vi "GSE 350 Read Data.vi"(8 "error in (no error)":errorcluster, 11 "VISA Refnum in":refnum<visa-resource-name>) -> (0 "error out":errorcluster, 2 "Raw Data":string, 3 "VISA Refnum out":refnum<visa-resource-name>)   [LabVIEW 2019]
uses:
  <vilib>/Utility/error.llb/whitespace.ctl
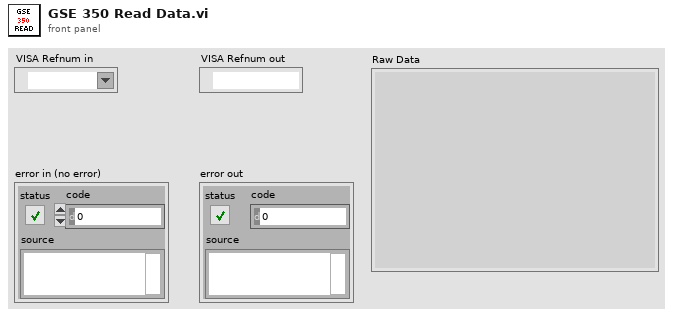
[diagram p1: front panel]
types:
  T1 = typedef "whitespace.ctl" = u16
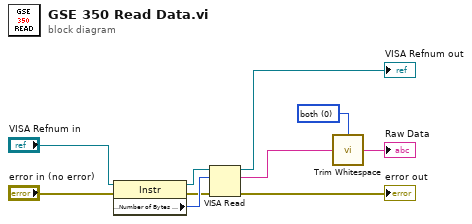
[diagram p0: block diagram]
diagram:
  w8 = T1 0 items=["both", "start of string", "end of string"] ("location (both)")
  n1 = property class="Instr"(reference="VISA Refnum in", error in="error in (no error)") -> (reference out=w4:refnum<visa-resource-name>, error out=w2:errorcluster, "Serial Settings:Number of Bytes at Serial Port"=w7:u32)
  n2 = VISA Read(VISA resource name=w4, byte count=w7, error in (no error)=w2) -> (VISA resource name out=→"VISA Refnum out":refnum<visa-resource-name>, read buffer=w9:string, error out=→"error out":errorcluster)  [unwired: 1 out]
  n3 = call <vilib>:"Trim Whitespace.vi"("string"=w9, "location (both)"=w8) -> ("trimmed string"=→"Raw Data":string)
